vi "initialise tasks.vi"(8 "error in (no error)":errorcluster, 11 "Waveform in":refnum<class "Waveform.lvclass">) -> (0 "error out":errorcluster, 3 "Waveform out":refnum<class "Waveform.lvclass">)   [LabVIEW 2012, in "Waveform.lvclass"]
uses:
  Waveform.lvclass
  Waveform.lvclass/Waveform.ctl
  <vilib>/DAQmx/write.llb/DAQmx Write (Analog DBL 1Chan 1Samp).vi
  <vilib>/DAQmx/write.llb/DAQmx Write (Digital 1D Bool 1Chan 1Samp).vi
  <vilib>/DAQmx/create/channels.llb/DAQmx Create Channel (AO-Voltage-Basic).vi
  <vilib>/DAQmx/create/channels.llb/DAQmx Create Channel (CO-Pulse Generation-Frequency).vi
  <vilib>/DAQmx/create/channels.llb/DAQmx Create Channel (DO-Digital Output).vi
  <vilib>/DAQmx/miscellaneous.llb/DAQmx Fill In Error Info.vi
  <resource>/objmgr/daqmx.rc
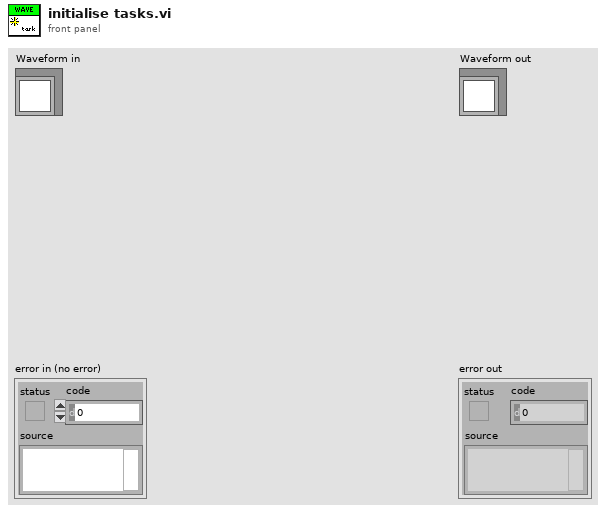
[diagram p1: front panel]
types:
  T1 = typedef "PC_wavelength.ctl" = dbl
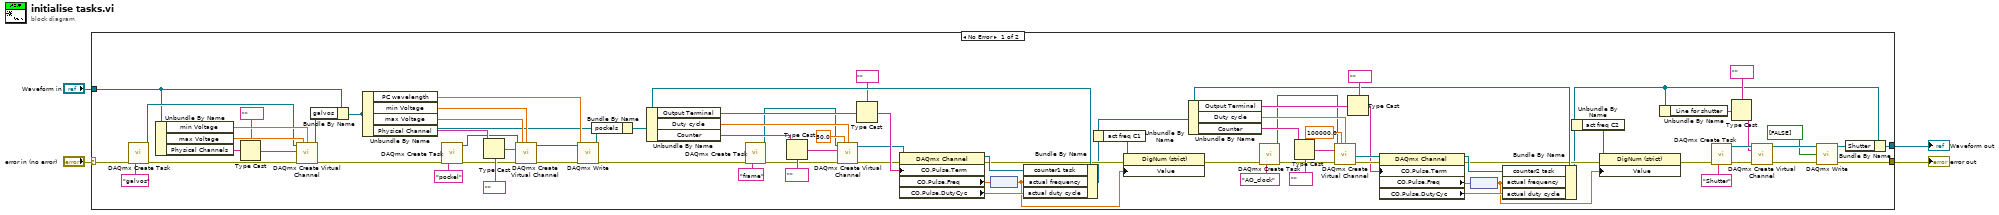
[diagram p0: block diagram]
diagram:
  n1 = case shown="No Error" "error in (no error)" {
    selector: "error in (no error)" -> [w29 w87]
    tunnel: [w10 w87] -> w3
    tunnel: [w6 w86] -> w1
    tunnel: "Waveform in" -> [w30 w86]
    frame No Error {
      n2 = call <vilib>:"DAQmx Create Task.vi"("new task name"="galvos", "error in"=w29) -> ("task out"=w44:refnum<k21>, "error out"=w46:errorcluster)  [unwired: 12 in]
      n3 = Unbundle By Name(w30) -> ("min Voltage"=w84:dbl, "max Voltage"=w85:dbl, "Physical Channels"=w68:string)
      n4 = Type Cast(type=tag "" ("physical channels"), x=w68) -> (*(type *) &x=w47:tag)
      n5 = call-poly <vilib>:"DAQmx Create Virtual Channel.vi"("task in"=w44, "maximum value"=w85, "minimum value"=w84, "physical channels"=w47, "error in"=w46) -> ("task out"=w27:refnum<k21>, "error out"=w28:errorcluster)  [unwired: 9 in]
      n6 = Bundle By Name(cluster=w30, "galvos"=w27) -> (w33:refnum<class "Waveform.lvclass">)
      n7 = Unbundle By Name(w33) -> ("PC wavelength"=w71:T1, "min Voltage"=w72:dbl, "max Voltage"=w73:dbl, "Physical Channel"=w66:string)
      n8 = call <vilib>:"DAQmx Create Task.vi"("new task name"="pockel", "error in"=w28) -> ("task out"=w42:refnum<k21>, "error out"=w43:errorcluster)  [unwired: 12 in]
      n9 = Type Cast(type=tag "" ("physical channels"), x=w66) -> (*(type *) &x=w65:tag)
      n10 = call-poly <vilib>:"DAQmx Create Virtual Channel.vi"("task in"=w42, "maximum value"=w73, "minimum value"=w72, "physical channels"=w65, "error in"=w43) -> ("task out"=w32:refnum<k21>, "error out"=w31:errorcluster)  [unwired: 9 in]
      n11 = call-poly <vilib>:"DAQmx Write.vi"("task/channels in"=w32, "data"=w71, "error in"=w31) -> ("task out"=w69:refnum<k21>, "error out"=w40:errorcluster)  [unwired: 10 in, 1 out]
      n12 = Bundle By Name(cluster=w33, "pockels"=w69) -> (w70:refnum<class "Waveform.lvclass">)
      n13 = Unbundle By Name(w70) -> ("Output Terminal"=w59:string, "Duty cycle"=w83:dbl, "Counter"=w63:string)
      n14 = call <vilib>:"DAQmx Create Task.vi"("new task name"="frame", "error in"=w40) -> ("task out"=w38:refnum<k21>, "error out"=w39:errorcluster)  [unwired: 12 in]
      n15 = Type Cast(type=tag "" ("counter"), x=w63) -> (*(type *) &x=w62:tag)
      n16 = call-poly <vilib>:"DAQmx Create Virtual Channel.vi"("task in"=w38, "frequency"=50.0, "duty cycle"=w83, "counter"=w62, "error in"=w39) -> ("task out"=w51:refnum<k21>, "error out"=w50:errorcluster)  [unwired: 9 in]
      n17 = Type Cast(type=tag "" ("CO.Pulse.Term"), x=w59) -> (*(type *) &x=w58:tag)
      n18 = property class="DAQmx Channel"(reference=w51, error in=w50, "CO.Pulse.Term"=w58) -> (reference out=w82:refnum<k21>, error out=w26:errorcluster, "CO.Pulse.Freq"=w81:dbl, "CO.Pulse.DutyCyc"=w80:dbl)
      n19 = node(w81) -> (w22:dbl[unit])
      n20 = Bundle By Name(cluster=w70, "counter1 task"=w82, "actual frequency"=w22, "actual duty cycle"=w80) -> (w24:refnum<class "Waveform.lvclass">)
      n21 = Unbundle By Name(w24) -> ("act freq C1"=w23:refnum<vi>)
      n22 = property class="DigNum (strict)"(reference=w23, error in=w26, "Value"=w22) -> (error out=w25:errorcluster)  [unwired: 1 out]
      n23 = Unbundle By Name(w24) -> ("Output Terminal"=w57:string, "Duty cycle"=w74:dbl, "Counter"=w54:string)
      n24 = call <vilib>:"DAQmx Create Task.vi"("new task name"="AO_clock", "error in"=w25) -> ("task out"=w35:refnum<k21>, "error out"=w36:errorcluster)  [unwired: 12 in]
      n25 = Type Cast(type=tag "" ("counter"), x=w54) -> (*(type *) &x=w52:tag)
      n26 = call-poly <vilib>:"DAQmx Create Virtual Channel.vi"("task in"=w35, "frequency"=100000.0, "duty cycle"=w74, "counter"=w52, "error in"=w36) -> ("task out"=w76:refnum<k21>, "error out"=w75:errorcluster)  [unwired: 9 in]
      n27 = Type Cast(type=tag "" ("CO.Pulse.Term"), x=w57) -> (*(type *) &x=w56:tag)
      n28 = property class="DAQmx Channel"(reference=w76, error in=w75, "CO.Pulse.Term"=w56) -> (reference out=w77:refnum<k21>, error out=w21:errorcluster, "CO.Pulse.Freq"=w78:dbl, "CO.Pulse.DutyCyc"=w79:dbl)
      n29 = node(w78) -> (w19:dbl[unit])
      n30 = Bundle By Name(cluster=w24, "counter2 task"=w77, "actual frequency"=w19, "actual duty cycle"=w79) -> (w7:refnum<class "Waveform.lvclass">)
      n31 = Unbundle By Name(w7) -> ("act freq C2"=w20:refnum<vi>)
      n32 = property class="DigNum (strict)"(reference=w20, error in=w21, "Value"=w19) -> (error out=w18:errorcluster)  [unwired: 1 out]
      n33 = Unbundle By Name(w7) -> ("Line for shutter"=w14:string)
      n34 = call <vilib>:"DAQmx Create Task.vi"("new task name"="Shutter", "error in"=w18) -> ("task out"=w15:refnum<k21>, "error out"=w16:errorcluster)  [unwired: 12 in]
      n35 = Type Cast(type=tag "" ("lines"), x=w14) -> (*(type *) &x=w12:tag)
      n36 = call-poly <vilib>:"DAQmx Create Virtual Channel.vi"("task in"=w15, "lines"=w12, "error in"=w16) -> ("task out"=w9:refnum<k21>, "error out"=w11:errorcluster)  [unwired: 11 in]
      n37 = call-poly <vilib>:"DAQmx Write.vi"("task/channels in"=w9, "data"=bool[] [FALSE], "error in"=w11) -> ("task out"=w5:refnum<k21>, "error out"=w10:errorcluster)  [unwired: 10 in, 1 out]
      n38 = Bundle By Name(cluster=w7, "Shutter"=w5) -> (w6:refnum<class "Waveform.lvclass">)
    }
    frame Error {
    }
  }
  "error out" <- w3
  "Waveform out" <- w1
